vi "GetExternalInterfaces.vi"(8 "Error In":errorcluster, 11 "reference in":refnum<class "MasterGUI.lvclass">) -> (0 "Error Out":errorcluster, 2 "ExternalInterfaces":T1[](array[typedef]), 3 "reference out":refnum<class "MasterGUI.lvclass">)   [LabVIEW 2021, in "MasterGUI.lvclass"]
uses:
  MasterGUI.lvclass
  Library_TAF_Support/ClusterArrayConversion/BundledArray.ctl
  Interface_TAF_ITAFObject/ITAFObject/ITAFObject.lvclass
  Library_TAF_Support/ClusterArrayConversion/ClusterArrayConversion.lvlib
  ec6bb0d8-241c-4bf6-bd1f-df29f73ad419.vi
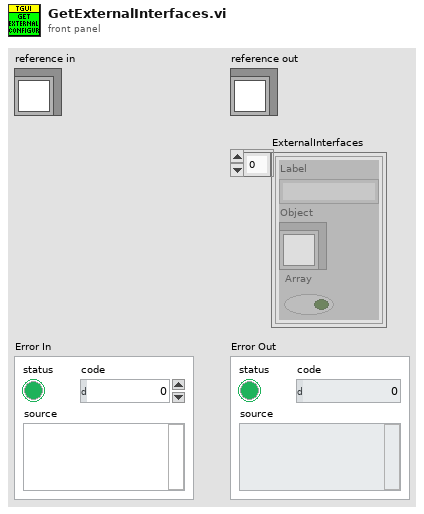
[diagram p1: front panel]
types:
  T1 = typedef "ClusterArrayConversion.lvlib/BundledArray.ctl" = cluster{"Label":string, "Object":refnum<class>, "Array":bool}
  T2 = typedef "MasterGUI.lvclass/ObjectAttributes.ctl" = cluster{"Interfaces":cluster{"dummy":refnum<class>}, "Locals":cluster{"MainGUIActive":refnum<queue>, "MainPanel":refnum<vi>, "LayoutPanel":cluster{"PanelVIRef":refnum<vi>, "Labels":string[], "SubPanels":refnum<vi>[]}, "MenuTree":T3[], "Menu":refnum<k9>}, "Persistent":cluster{"StaticDocking":cluster{"ObjectLabel":string, "SubPanelLabel":string}[], "WindowsTitle":string, "AdditionalMenuItems":T3[], "TraceObjectName":string}}
  T3 = typedef "MasterGUI.lvclass/MenuItem.ctl" = cluster{"Parent":string, "Items":string[], "ShortCuts":cluster{"IncludeShiftKey":bool, "IncludeCtrlKey":bool, "ShortcutKey":string}[]}
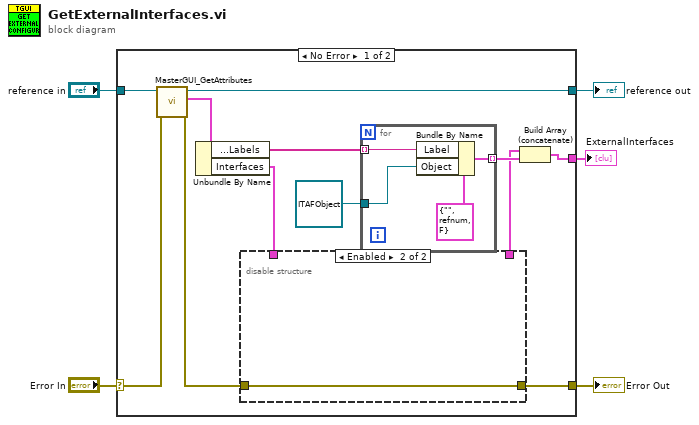
[diagram p0: block diagram]
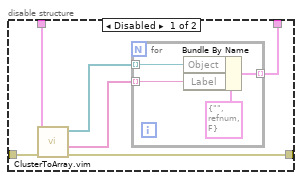
[diagram p2: hidden frame]
diagram:
  n1 = case shown="No Error" "Error In" {
    selector: "Error In" -> [w17 w34]
    tunnel: [w9 w34] -> w4
    tunnel: [w14 w33] -> w2
    tunnel: "reference in" -> [w15 w33]
    tunnel: [w7 _] -> w1
    frame No Error {
      n2 = call "MasterGUI_GetAttributes.vi"("error in (no error)"=w17, "reference in"=w15) -> ("error out"=w10:errorcluster, "Data"=w16:T2, "reference out"=w14:refnum<class "MasterGUI.lvclass">)  [unwired: 6 in, 1 out]
      n3 = Unbundle By Name(w16) -> ("Locals.LayoutPanel.Labels"=w13:string[], "Interfaces"=w8:cluster{"dummy":refnum<class>})
      n4 = disable-structure shown="Enabled" {
        disable-tunnel: w10 -> [w23 w28]
        disable-tunnel: [w22 w28] -> w9
        disable-tunnel: w8 -> [w21 _]
        disable-tunnel: [w18 _] -> w6
        frame Disabled {
          n5 = call "ClusterToArray.vim"("Error In"=w23, "Cluster"=w21) -> ("Error Out"=w22:errorcluster, "Labels"=w19:string[], "ArrayOfElements"=w20:refnum<class>[])  [unwired: 7 in]
          n6 = for {
            tunnel: w20 -> [w26] mode=indexing
            tunnel: w19 -> [w25] mode=indexing
            tunnel: [w24] -> w18 mode=indexing
            n7 = Bundle By Name(cluster=T1 {"Label"="", "Object"=refnum, "Array"=FALSE} ("ExternalInterface"), "Object"=w26, "Label"=w25) -> (w24:T1)
          }
        }
        frame Enabled {
        }
      }
      n8 = for {
        tunnel: w13 -> [w31] mode=indexing
        tunnel: refnum<class "ITAFObject.lvclass"> refnum ("NamedCreator") -> [w30]
        tunnel: [w29] -> w11 mode=indexing
        n9 = Bundle By Name(cluster=T1 {"Label"="", "Object"=refnum, "Array"=FALSE} ("ExternalInterface"), "Label"=w31, "Object"=w30) -> (w29:T1)
      }
      n10 = Build Array (concatenate)(w6, w11) -> (w7:T1[])
    }
    frame Error {
    }
  }
  "Error Out" <- w4
  "reference out" <- w2
  "ExternalInterfaces" <- w1
